vi "有效负载布放与回收.vi"() -> ()   [LabVIEW 2018]
uses:
  D:/Labview2018/examples/Instrument IO/Serial/support/Serial - Settings.ctl
  <vilib>/Instr/_visa.llb/VISA Configure Serial Port (Instr).vi
  <vilib>/Utility/inputDevices.llb/closeJoystick.vi
panel:
  in  "选项卡控件 8":T1(tab)
  out "潜航器模式":i32
  out "潜航器速度":i32
  out "悬停":bool
  out "定深":bool
  out "定向":bool
  in  "VISA资源名称":refnum<visa-resource-name>="COM1"
  in  "串口设置":T2={"波特率"=9600, "数据位"=8, "校验"=enum."None", "停止位"=10, "流控制"=0} {"流控制" items=["无"=0, "XON/XOFF"=1, "RTS/CTS"=2, "DTR/DSR"=4]; "停止位" items=["1.0"=10, "1.5"=15, "2.0"=20]; "数据位" min=5 max=8 step=1; "波特率" items=["75"=75, "110"=110, "134"=134, "150"=150, "300"=300, "600"=600, "1200"=1200, "1800"=1800, "2400"=2400, "4800"=4800, "7200"=7200, "9600"=9600, "14400"=14400, "19200"=19200, "28800"=28800, "38400"=38400, "56000"=56000, "57600"=57600, "115200"=115200, "128000"=128000, "230400"=230400]}
  out "指示灯":cluster{bool, bool, bool}
  out "位置信息":cluster{dbl, dbl}
  out "Polar Plot":picture caption="极坐标图"
  out "显示界面":T3
  out "桅杆升到位":bool
  out "桅杆降到位":bool
  out "挡板缸":bool
  out "俯仰缸":bool
  out "升降桅杆缸":bool
  out "仰到位":bool
  out "俯到位":bool
  out "挡板张开到位":bool
  out "挡板合拢到位":bool
  in  "停止":bool
  out "俯仰位移传感器":i64 caption="Output Value"
  out "挡板推进传感器":i64 caption="Output Value"
  out "升降桅杆位移传感器":i64 caption="Output Value"
  out "系统通讯故障":bool
  out "系统通讯正常":bool
  in  "照明灯":bool
  in  "停止 2":bool
  in  "抱紧 2":bool
  in  "打开 2":bool
  out "推进模块故障":bool caption="地位正常运行"
  out "推进模块正常":bool
  out "推进模块故障信息":string
  out "电机运行状态":bool
  out "未到位":bool
  out "缩回到位":bool
  out "推进到位":bool
  out "Output Value 18":dbl caption="Output Value" format="%.2f"
  out "Output Value 17":dbl caption="Output Value" format="%.2f"
  out "Output Value 16":dbl caption="Output Value" format="%.2f"
  out "Output Value 15":dbl caption="Output Value" format="%.2f"
  out "Output Value 14":dbl caption="Output Value" format="%.2f"
  out "Output Value 13":dbl caption="Output Value" format="%.2f"
  out "Output Value 12":dbl caption="Output Value" format="%.2f"
  out "Output Value 11":dbl caption="Output Value" format="%.2f"
  out "Output Value 10":dbl caption="Output Value" format="%.2f"
  out "Output Value 9":dbl caption="Output Value" format="%.2f"
  out "Output Value 8":dbl caption="Output Value" format="%.2f"
  out "Output Value 7":dbl caption="Output Value" format="%.2f"
  out "Output Value 6":dbl caption="Output Value" format="%.2f"
  out "Output Value 5":dbl caption="Output Value" format="%.2f"
  out "Output Value 4":dbl caption="Output Value" format="%.2f"
  out "Output Value 3":dbl caption="Output Value" format="%.2f"
  out "Output Value 2":dbl caption="Output Value" format="%.2f"
  out "Output Value":dbl format="%.2f"
  in  "Application filename":string="canceshi1"
  in  "IP Port":string="22222"
  in  "IP Address":string="192.168.0.10"
  out "旋转":dbl caption="Output Value" format="%.2f"
  out "升降":dbl caption="Output Value" format="%.2f"
  out "抱爪1":dbl caption="Output Value" format="%.2f"
  out "伺服阀":dbl caption="Output Value" format="%.2f"
  in  "停止":bool
  in  "抱紧":bool
  in  "打开":bool
  out "电机2运行状态":bool
  out "抱爪2未到位":bool
  out "抱爪2抱紧到位":bool
  out "抱爪2打开到位":bool
  out "电机1运行状态":bool
  out "抱爪1未到位":bool
  out "抱爪1抱紧到位":bool
  out "抱爪1打开到位":bool
  out "电机2或驱动器2故障":bool
  out "电机2或驱动器2正常":bool
  out "电机1或驱动器1故障":bool
  out "电机1或驱动器1正常":bool
  out "回转故障信息":string
  in  "停止 3":bool
  in  "原始位":bool
  in  "工作位":bool
  out "到达工作位":bool
  out "电机运行状态":bool
  out "未到位":bool
  out "到达原始位":bool
  out "回转模块故障":bool caption="地位正常运行"
  out "回转模块正常":bool
  # "单位/mm"
  # "单位/mm"
  # "单位/mm"
  # "推进控制模块"
  # "捕获臂控制模块"
  # "回转控制模块"
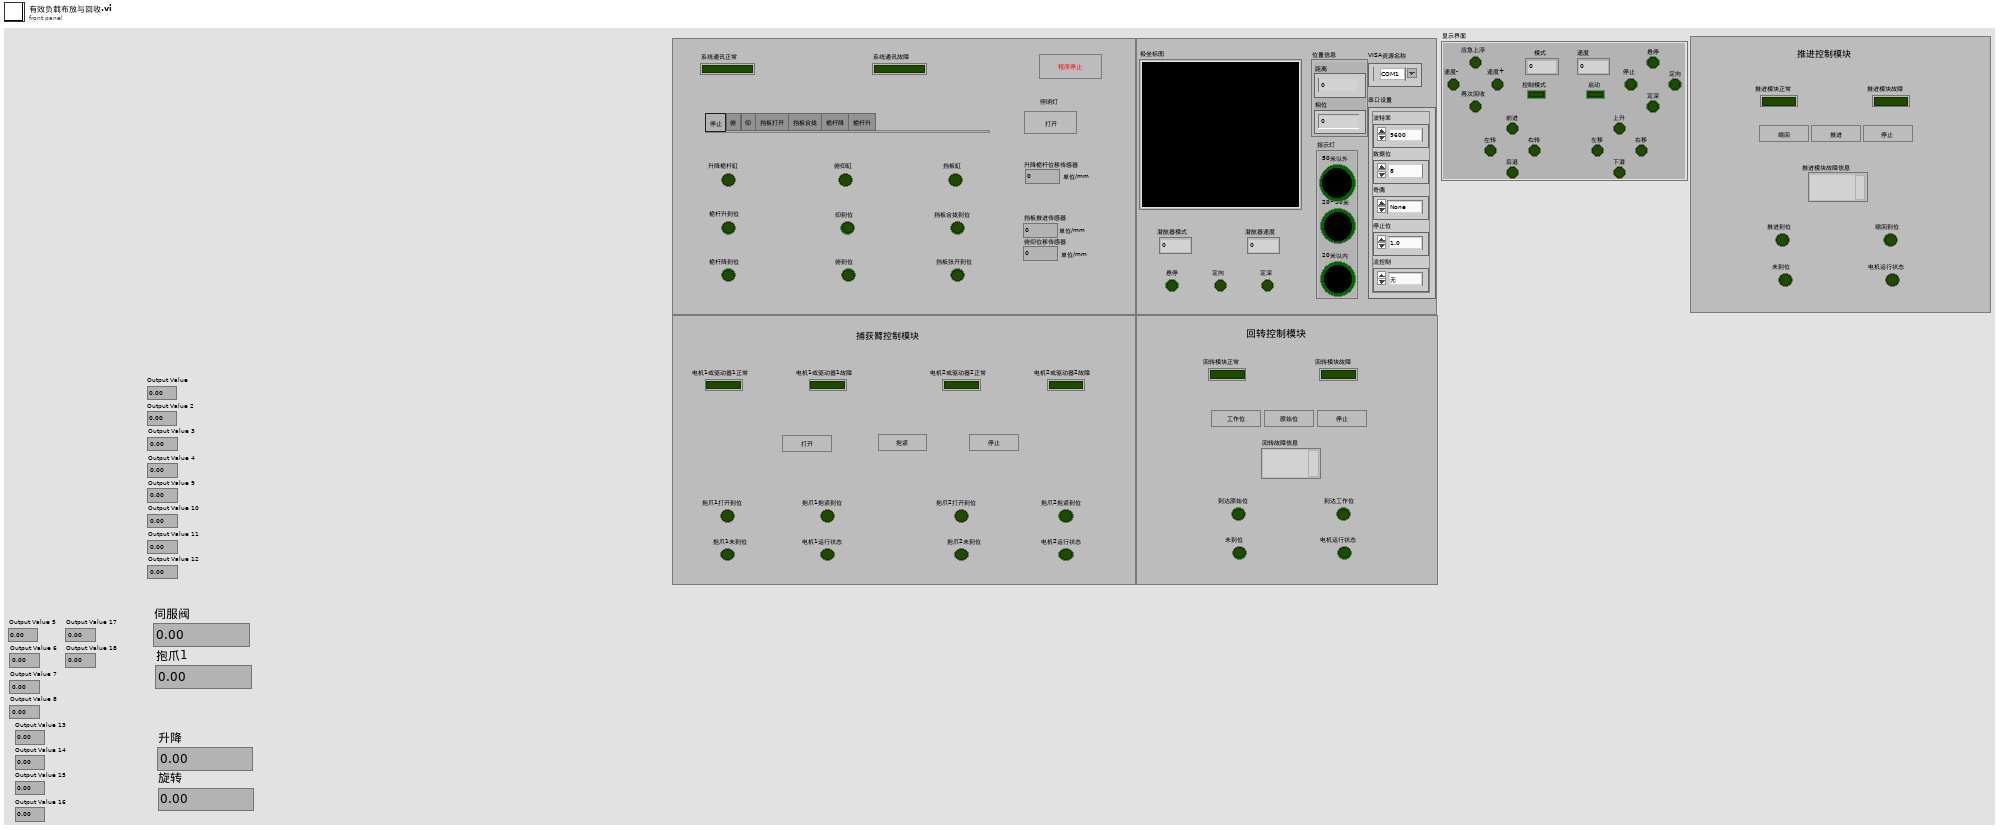
[diagram p1: front panel]
types:
  T1 = enum32{"停止", "俯", "仰", "挡板打开", "挡板合拢", "桅杆降", "桅杆升"}
  T2 = typedef "Serial - Settings.ctl" = cluster{"波特率":u32, "数据位":u16, "校验":enum16{"None", "Odd", "Even", "Mark", "Space"}, "停止位":u16, "流控制":u16}
  T3 = cluster{"右转":bool, "左转":bool, "后退":bool, "前进":bool, "右移":bool, "左移":bool, "下潜":bool, "上升":bool, "定深":bool, "定向":bool, "停止":bool, "悬停":bool, "控制模式":bool, "启动":bool, "应急上浮":bool, "再次回收":bool, "速度+":bool, "速度-":bool, "模式":i32, "速度":i32}
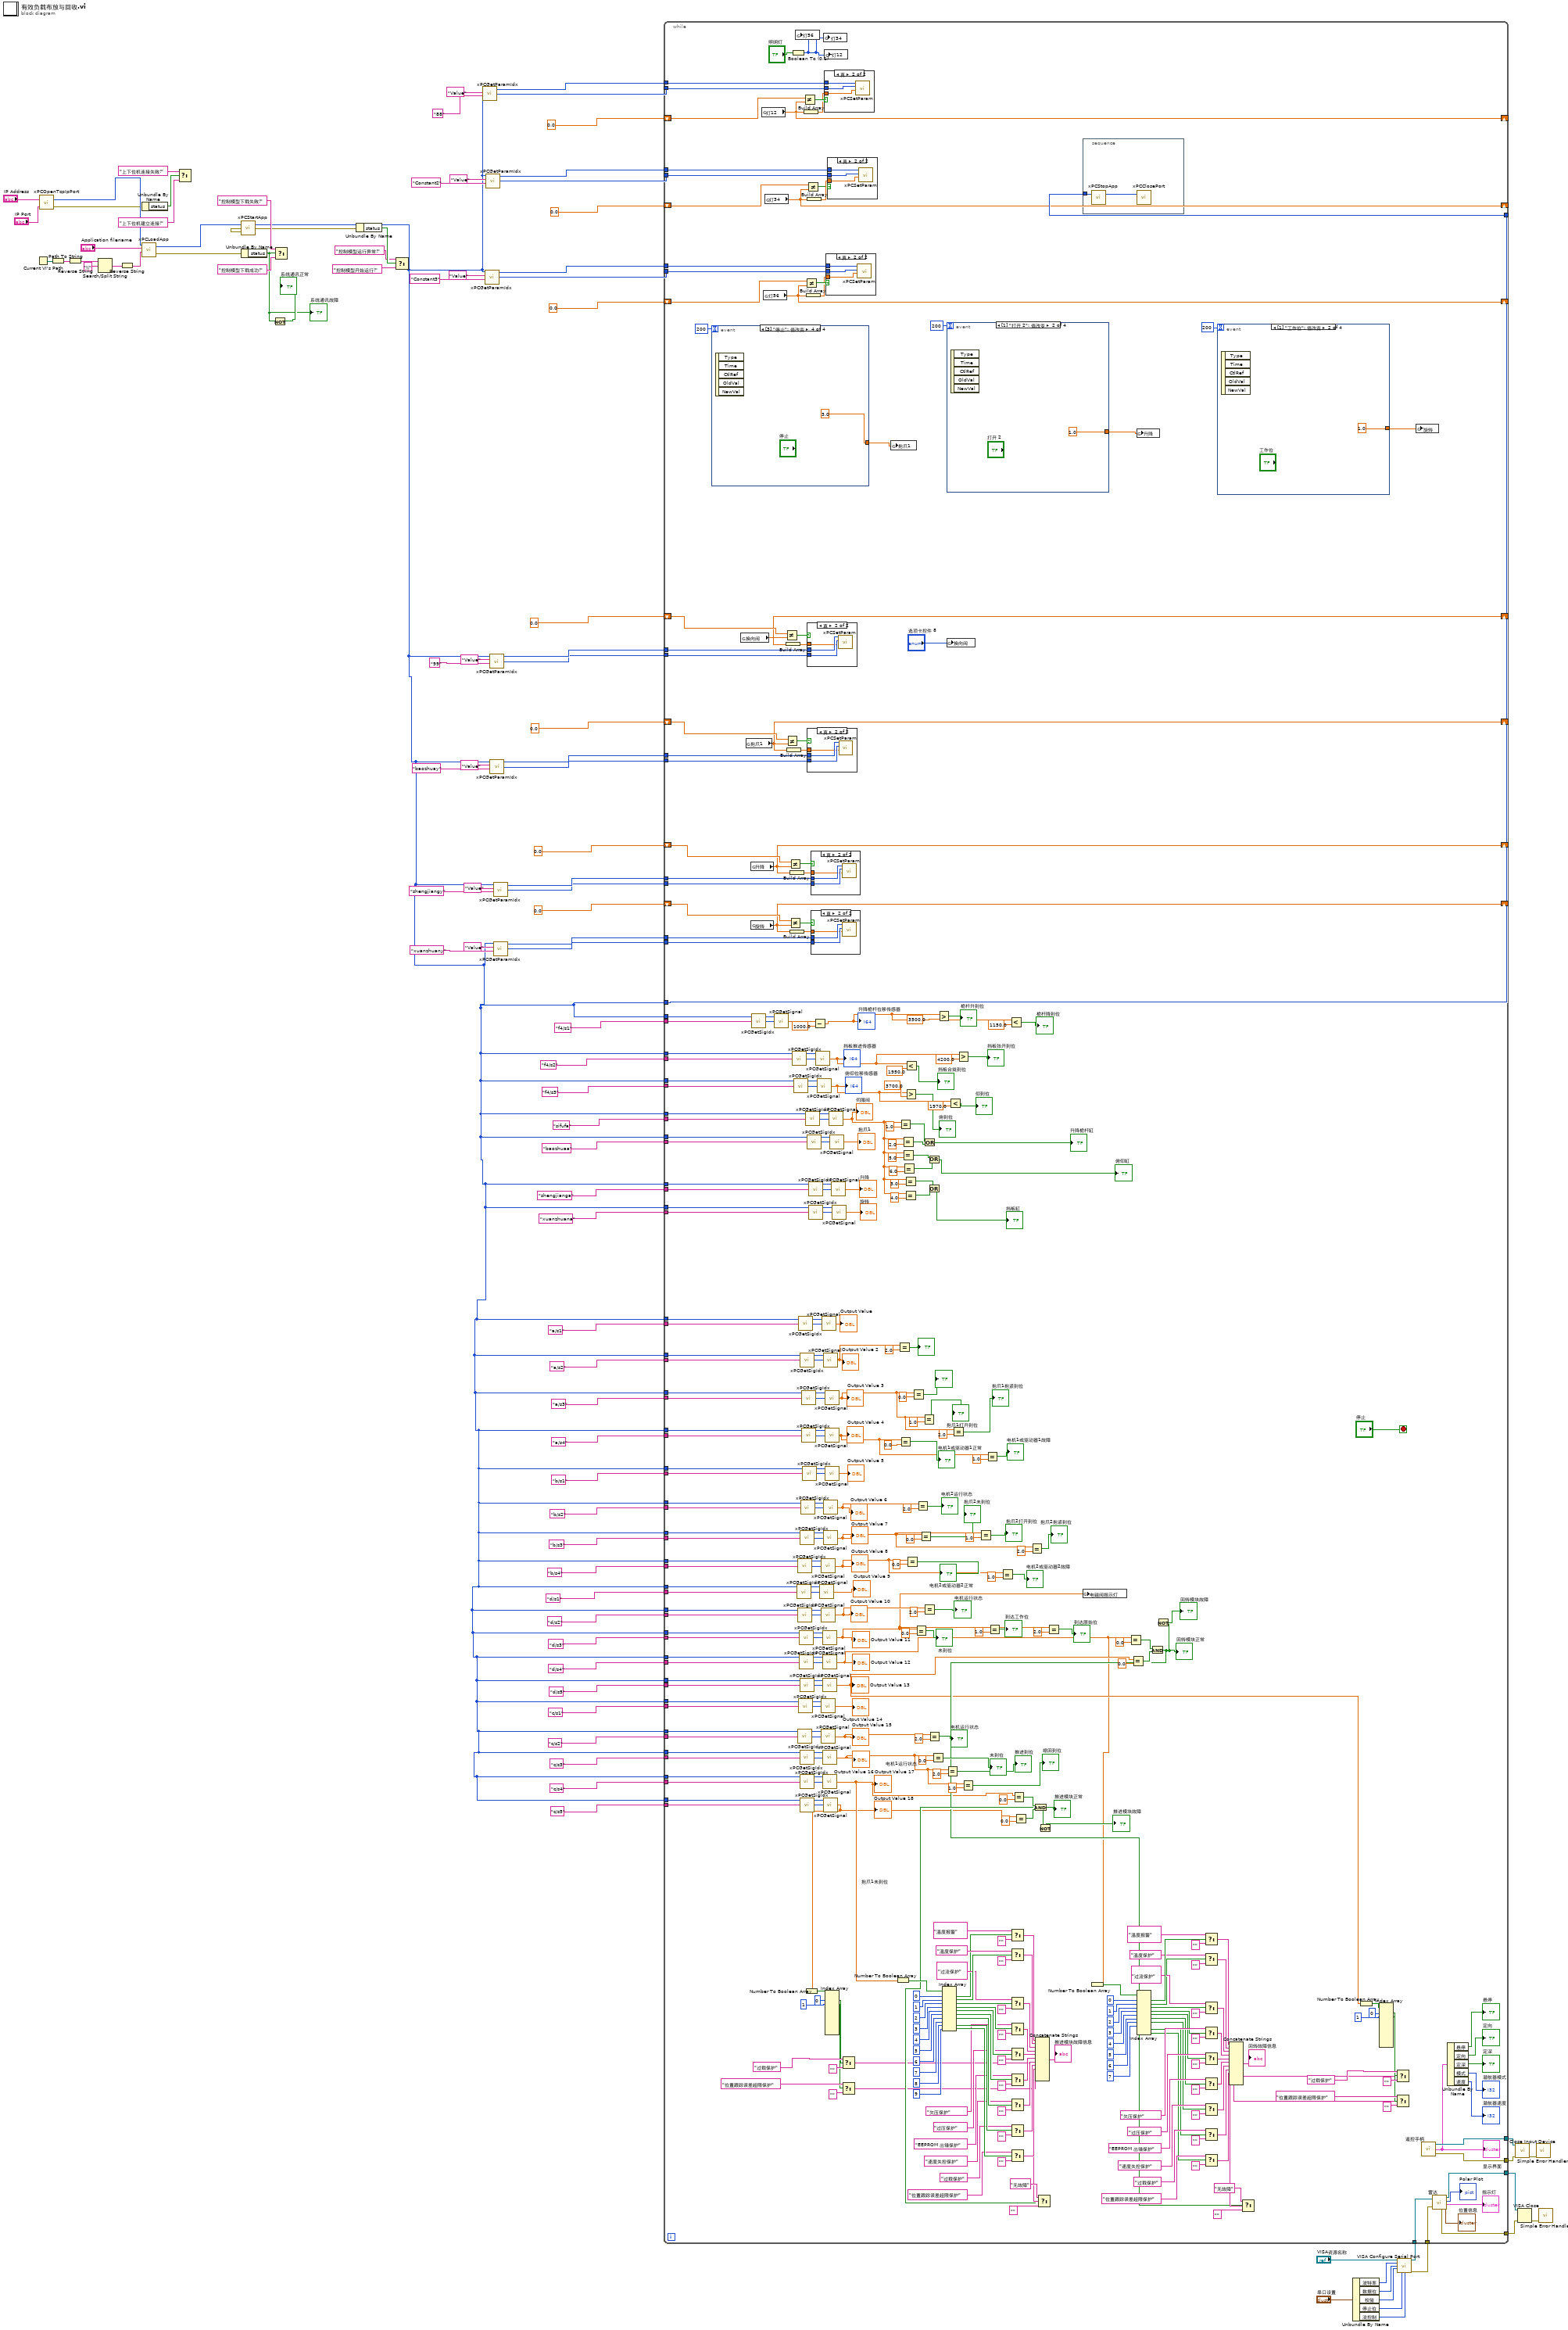
[diagram p0: block diagram]
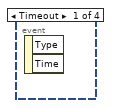
[diagram p2: hidden frame]
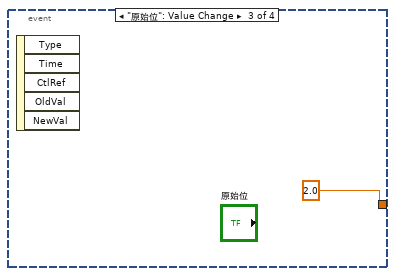
[diagram p3: hidden frame]
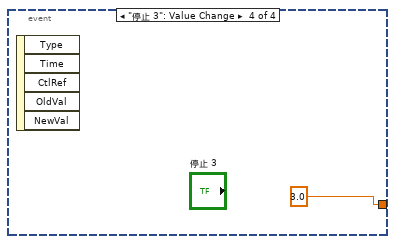
[diagram p4: hidden frame]
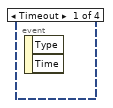
[diagram p5: hidden frame]
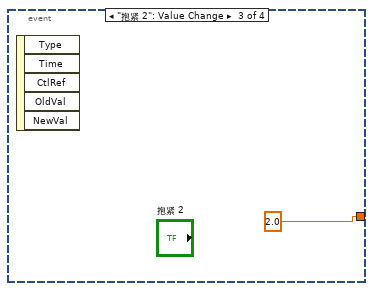
[diagram p6: hidden frame]
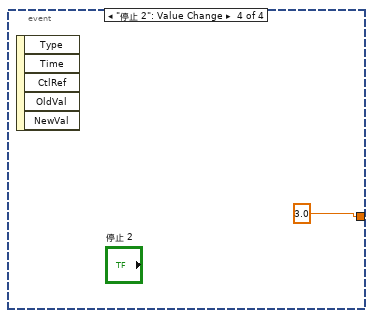
[diagram p7: hidden frame]
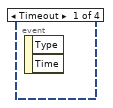
[diagram p8: hidden frame]
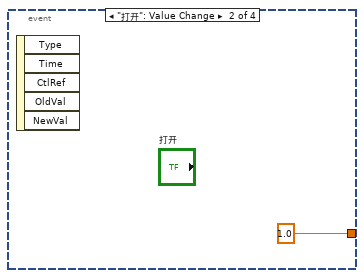
[diagram p9: hidden frame]
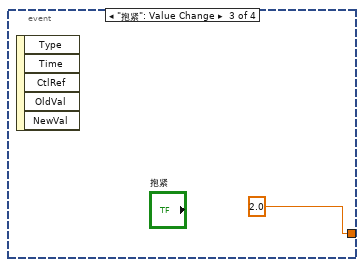
[diagram p10: hidden frame]
diagram:
  n1 = Current VI's Path() -> (path=w95:path)
  n2 = call "xPCOpenTcpIpPort.vi"("port"="IP Port", "address"="IP Address") -> ("error out"=w85:errorcluster, "Port"=w86:i32)
  n3 = Path To String(path=w95) -> (string=w97:string)
  n4 = Reverse String(1:w97) -> (0:w99:string)
  n5 = Search/Split String(string=w99, search string/char (-)="\\" ("search char (-)")) -> (match + rest of string=w98:string)  [unwired: 1 in, 2 out]
  n6 = Reverse String(1:w98) -> (0:w100:string)
  n7 = Unbundle By Name(w85) -> ("status"=w92:bool)
  n8 = call "xPCLoadApp.vi"("pathstr"=w100, "filename"="Application filename", "port"=w86) -> ("error out"=w87:errorcluster, "port copy"=w94:i32)  [unwired: 1 in]
  n9 = Select(t="上下位机连接失败!" ("message"), s=w92, f="上下位机建立连接!" ("message")) -> ()  [unwired: 1 out]
  n10 = call "xPCStartApp.vi"("port"=w94) -> ("error out"=w79:errorcluster, "port copy"=w16:i32)  [unwired: 1 in]
  n11 = Unbundle By Name(w87) -> ("status"=w52:bool)
  "系统通讯故障" <- w52
  n12 = Not(x=w52) -> (.not. x?=→"系统通讯正常":bool)
  n13 = Select(t="控制模型下载失败!" ("message"), s=w52, f="控制模型下载成功!" ("message")) -> ()  [unwired: 1 out]
  n14 = Unbundle By Name(w79) -> ("status"=w81:bool)
  n15 = Select(t="控制模型运行异常!" ("message"), s=w81, f="控制模型开始运行!" ("message")) -> ()  [unwired: 1 out]
  n16 = call "xPCGetParamIdx.vi"("blockpath"="88" ("pathstr"), "parametername"="Value" ("filename"), "port"=w16) -> ("identifier"=w72:i32, "port copy"=w73:i32)  [unwired: 1 in, 1 out]
  n17 = call "xPCGetParamIdx.vi"("blockpath"="Constant3" ("pathstr"), "parametername"="Value" ("filename"), "port"=w16) -> ("identifier"=w61:i32, "port copy"=w62:i32)  [unwired: 1 in, 1 out]
  n18 = call "xPCGetParamIdx.vi"("blockpath"="Constant2" ("pathstr"), "parametername"="Value" ("filename"), "port"=w16) -> ("identifier"=w66:i32, "port copy"=w65:i32)  [unwired: 1 in, 1 out]
  n19 = call "xPCGetParamIdx.vi"("blockpath"="99" ("pathstr"), "parametername"="Value" ("filename"), "port"=w16) -> ("identifier"=w58:i32, "port copy"=w76:i32)  [unwired: 1 in, 1 out]
  n20 = call "xPCGetParamIdx.vi"("blockpath"="baozhuay" ("pathstr"), "parametername"="Value" ("filename"), "port"=w16) -> ("identifier"=w31:i32, "port copy"=w29:i32)  [unwired: 1 in, 1 out]
  n21 = call "xPCGetParamIdx.vi"("blockpath"="shengjiangy" ("pathstr"), "parametername"="Value" ("filename"), "port"=w16) -> ("identifier"=w22:i32, "port copy"=w24:i32)  [unwired: 1 in, 1 out]
  n22 = call "xPCGetParamIdx.vi"("blockpath"="xuanzhuany" ("pathstr"), "parametername"="Value" ("filename"), "port"=w16) -> ("identifier"=w21:i32, "port copy"=w19:i32)  [unwired: 1 in, 1 out]
  n23 = Unbundle By Name("串口设置") -> ("波特率"=w7:u32, "数据位"=w8:u16, "校验"=w9:enum16{"None", "Odd", "Even", "Mark", "Space"}, "停止位"=w10:u16, "流控制"=w5:u16)
  n24 = call-poly "VISA Configure Serial Port"("VISA resource name"="VISA资源名称", "baud rate (9600)"=w7, "data bits (8)"=w8, "parity (0:none)"=w9, "stop bits (10: 1 bit)"=w10, "flow control (0:none)"=w5) -> ("VISA resource name out"=w4:refnum<visa-resource-name>, "error out"=w3:errorcluster)  [unwired: 4 in, 4 out]
  n25 = while {
    tunnel: w16 -> [w497]
    tunnel: [w497] -> w93
    shift-right: [w491] -> _
    shift-left: 0.0 -> [w494]
    tunnel: w58 -> [w493]
    tunnel: w76 -> [w492]
    shift-right: [w490] -> _
    shift-left: 0.0 -> [w489]
    tunnel: w72 -> [w486]
    tunnel: w73 -> [w485]
    tunnel: w16 -> [w483]
    tunnel: "f4/s1" ("pathstr") -> [w481]
    shift-right: [w474] -> _
    shift-left: 0.0 -> [w475]
    tunnel: w66 -> [w478]
    tunnel: w65 -> [w479]
    shift-right: [w473] -> _
    shift-left: 0.0 -> [w472]
    tunnel: w61 -> [w469]
    tunnel: w62 -> [w468]
    tunnel: w16 -> [w464]
    tunnel: "sifufa" ("pathstr") -> [w466]
    tunnel: w16 -> [w463]
    tunnel: "baozhuaa" ("pathstr") -> [w460]
    tunnel: w16 -> [w458]
    tunnel: "shengjianga" ("pathstr") -> [w455]
    tunnel: w16 -> [w449]
    tunnel: "xuanzhuana" ("pathstr") -> [w452]
    tunnel: w16 -> [w424]
    tunnel: "a/s1" ("pathstr") -> [w422]
    tunnel: w16 -> [w425]
    tunnel: "a/s2" ("pathstr") -> [w427]
    tunnel: w16 -> [w432]
    tunnel: "a/s3" ("pathstr") -> [w430]
    tunnel: w16 -> [w433]
    tunnel: "a/s4" ("pathstr") -> [w435]
    tunnel: w16 -> [w440]
    tunnel: "b/s1" ("pathstr") -> [w438]
    tunnel: w16 -> [w441]
    tunnel: "b/s2" ("pathstr") -> [w443]
    tunnel: w16 -> [w448]
    tunnel: "b/s3" ("pathstr") -> [w446]
    tunnel: w16 -> [w420]
    tunnel: "b/s4" ("pathstr") -> [w418]
    tunnel: w16 -> [w413]
    tunnel: "d/s1" ("pathstr") -> [w415]
    tunnel: w16 -> [w412]
    tunnel: "d/s2" ("pathstr") -> [w410]
    tunnel: w16 -> [w405]
    tunnel: "d/s3" ("pathstr") -> [w407]
    tunnel: w16 -> [w404]
    tunnel: "d/s4" ("pathstr") -> [w402]
    tunnel: w16 -> [w397]
    tunnel: "d/s5" ("pathstr") -> [w399]
    tunnel: w16 -> [w396]
    tunnel: "c/s1" ("pathstr") -> [w394]
    tunnel: w16 -> [w389]
    tunnel: "c/s2" ("pathstr") -> [w391]
    tunnel: w16 -> [w380]
    tunnel: "c/s3" ("pathstr") -> [w378]
    tunnel: w16 -> [w381]
    tunnel: "c/s4" ("pathstr") -> [w383]
    tunnel: w16 -> [w388]
    tunnel: "c/s5" ("pathstr") -> [w386]
    tunnel: w16 -> [w220]
    tunnel: "f4/s2" ("pathstr") -> [w222]
    tunnel: w16 -> [w219]
    tunnel: "f4/s3" ("pathstr") -> [w217]
    shift-right: [w161] -> _
    shift-left: 0.0 -> [w174]
    tunnel: w31 -> [w175]
    tunnel: w29 -> [w176]
    shift-right: [w160] -> _
    shift-left: 0.0 -> [w169]
    tunnel: w22 -> [w168]
    tunnel: w24 -> [w167]
    shift-right: [w159] -> _
    shift-left: 0.0 -> [w164]
    tunnel: w21 -> [w165]
    tunnel: w19 -> [w166]
    tunnel: [w117] -> w14
    tunnel: [w116] -> w13
    tunnel: w4 -> [w112]
    tunnel: w3 -> [w111]
    tunnel: [w110] -> w2
    tunnel: [w109] -> w1
    stop <- "停止" stop-if-true
    n26 = event shown="[3] \"停止\": 值改变" {
      selector: _ -> [_ _ _ _]
      dyn-events: _ -> [_ _ _ _]
      timeout: 200 -> [_ _ _ _]
      tunnel: [_ 1.0 ("抱爪1") 2.0 ("抱爪1") 3.0 ("抱爪1")] -> w157
      event Timeout {
        n27 = event-data() -> ()  [unwired: 1 in, 2 out]
      }
      event "打开": Value Change {
        n28 = event-data() -> ()  [unwired: 1 in, 5 out]
      }
      event "抱紧": Value Change {
        n29 = event-data() -> ()  [unwired: 1 in, 5 out]
      }
      event "停止": Value Change {
        n30 = event-data() -> ()  [unwired: 1 in, 5 out]
      }
    }
    n31 = global read "全局 1.vi" "换向阀"() -> (w491:dbl)
    n32 = global read "全局 1.vi" "抱爪1"() -> (w161:dbl)
    n33 = global read "全局 1.vi" "升降"() -> (w160:dbl)
    n34 = global read "全局 1.vi" "旋转"() -> (w159:dbl)
    n35 = call "xPCGetSigIdx.vi"("blockpath"=w481, "port"=w483) -> ("identifier"=w480:i32, "port copy"=w482:i32)  [unwired: 1 in, 1 out]
    n36 = global read "全局 1.vi" "灯12"() -> (w490:dbl)
    n37 = global read "全局 1.vi" "灯56"() -> (w473:dbl)
    n38 = global read "全局 1.vi" "灯34"() -> (w474:dbl)
    n39 = call "xPCGetSignal.vi"("signal"=w480, "port"=w482) -> ("Output Value"=w120:dbl)  [unwired: 1 in, 2 out]
    n40 = Not Equal?(x=w494, y=w491) -> (x != y?=w495:bool)
    n41 = Not Equal?(x=w174, y=w161) -> (x != y?=w173:bool)
    n42 = Build Array(w491) -> (w496:dbl[])
    n43 = Build Array(w161) -> (w172:dbl[])
    n44 = Not Equal?(x=w169, y=w160) -> (x != y?=w170:bool)
    n45 = Not Equal?(x=w164, y=w159) -> (x != y?=w163:bool)
    n46 = Build Array(w160) -> (w171:dbl[])
    n47 = Build Array(w159) -> (w162:dbl[])
    n48 = Boolean To (0,1)(Boolean="照明灯") -> (0, 1=w121:i16)
    n49 = call "xPCGetSigIdx.vi"("blockpath"=w222, "port"=w220) -> ("identifier"=w223:i32, "port copy"=w221:i32)  [unwired: 1 in, 1 out]
    n50 = call "xPCGetSigIdx.vi"("blockpath"=w217, "port"=w219) -> ("identifier"=w216:i32, "port copy"=w218:i32)  [unwired: 1 in, 1 out]
    n51 = global write "全局 1.vi" "灯56"(w121) -> ()
    n52 = call "xPCGetSigIdx.vi"("blockpath"=w415, "port"=w413) -> ("identifier"=w416:i32, "port copy"=w414:i32)  [unwired: 1 in, 1 out]
    n53 = call "xPCGetSigIdx.vi"("blockpath"=w418, "port"=w420) -> ("identifier"=w417:i32, "port copy"=w419:i32)  [unwired: 1 in, 1 out]
    n54 = call "xPCGetSigIdx.vi"("blockpath"=w410, "port"=w412) -> ("identifier"=w409:i32, "port copy"=w411:i32)  [unwired: 1 in, 1 out]
    n55 = call "xPCGetSigIdx.vi"("blockpath"=w391, "port"=w389) -> ("identifier"=w392:i32, "port copy"=w390:i32)  [unwired: 1 in, 1 out]
    n56 = call "xPCGetSigIdx.vi"("blockpath"=w394, "port"=w396) -> ("identifier"=w393:i32, "port copy"=w395:i32)  [unwired: 1 in, 1 out]
    n57 = call "xPCGetSigIdx.vi"("blockpath"=w422, "port"=w424) -> ("identifier"=w421:i32, "port copy"=w423:i32)  [unwired: 1 in, 1 out]
    n58 = call "xPCGetSigIdx.vi"("blockpath"=w407, "port"=w405) -> ("identifier"=w408:i32, "port copy"=w406:i32)  [unwired: 1 in, 1 out]
    n59 = call "xPCGetSigIdx.vi"("blockpath"=w402, "port"=w404) -> ("identifier"=w401:i32, "port copy"=w403:i32)  [unwired: 1 in, 1 out]
    n60 = call "xPCGetSigIdx.vi"("blockpath"=w399, "port"=w397) -> ("identifier"=w400:i32, "port copy"=w398:i32)  [unwired: 1 in, 1 out]
    n61 = call "xPCGetSigIdx.vi"("blockpath"=w378, "port"=w380) -> ("identifier"=w377:i32, "port copy"=w379:i32)  [unwired: 1 in, 1 out]
    n62 = call "xPCGetSigIdx.vi"("blockpath"=w383, "port"=w381) -> ("identifier"=w384:i32, "port copy"=w382:i32)  [unwired: 1 in, 1 out]
    n63 = call "xPCGetSigIdx.vi"("blockpath"=w427, "port"=w425) -> ("identifier"=w428:i32, "port copy"=w426:i32)  [unwired: 1 in, 1 out]
    n64 = call "xPCGetSigIdx.vi"("blockpath"=w446, "port"=w448) -> ("identifier"=w445:i32, "port copy"=w447:i32)  [unwired: 1 in, 1 out]
    n65 = call "xPCGetSigIdx.vi"("blockpath"=w386, "port"=w388) -> ("identifier"=w385:i32, "port copy"=w387:i32)  [unwired: 1 in, 1 out]
    n66 = call "xPCGetSigIdx.vi"("blockpath"=w443, "port"=w441) -> ("identifier"=w444:i32, "port copy"=w442:i32)  [unwired: 1 in, 1 out]
    n67 = call "xPCGetSigIdx.vi"("blockpath"=w430, "port"=w432) -> ("identifier"=w429:i32, "port copy"=w431:i32)  [unwired: 1 in, 1 out]
    n68 = call "xPCGetSigIdx.vi"("blockpath"=w435, "port"=w433) -> ("identifier"=w436:i32, "port copy"=w434:i32)  [unwired: 1 in, 1 out]
    n69 = call "xPCGetSigIdx.vi"("blockpath"=w438, "port"=w440) -> ("identifier"=w437:i32, "port copy"=w439:i32)  [unwired: 1 in, 1 out]
    n70 = Not Equal?(x=w489, y=w490) -> (x != y?=w488:bool)
    n71 = Build Array(w490) -> (w487:dbl[])
    n72 = Not Equal?(x=w472, y=w473) -> (x != y?=w471:bool)
    n73 = call "xPCGetSigIdx.vi"("blockpath"=w466, "port"=w464) -> ("identifier"=w467:i32, "port copy"=w465:i32)  [unwired: 1 in, 1 out]
    n74 = Not Equal?(x=w475, y=w474) -> (x != y?=w476:bool)
    n75 = Build Array(w473) -> (w470:dbl[])
    n76 = case shown="真" w495 {
      tunnel: w492 -> [_ w527]
      tunnel: w493 -> [_ w526]
      tunnel: w496 -> [_ w525]
      frame False {
      }
      frame True {
        n77 = call "xPCSetParam.vi"("value"=w525, "index"=w526, "port"=w527) -> ()  [unwired: 1 in, 2 out]
      }
    }
    n78 = call "xPCGetSigIdx.vi"("blockpath"=w460, "port"=w463) -> ("identifier"=w459:i32, "port copy"=w462:i32)  [unwired: 1 in, 1 out]
    n79 = Build Array(w474) -> (w477:dbl[])
    n80 = case shown="真" w173 {
      tunnel: w176 -> [_ w515]
      tunnel: w175 -> [_ w514]
      tunnel: w172 -> [_ w513]
      frame False {
      }
      frame True {
        n81 = call "xPCSetParam.vi"("value"=w513, "index"=w514, "port"=w515) -> ()  [unwired: 1 in, 2 out]
      }
    }
    n82 = call "xPCGetSigIdx.vi"("blockpath"=w455, "port"=w458) -> ("identifier"=w454:i32, "port copy"=w457:i32)  [unwired: 1 in, 1 out]
    n83 = call "xPCGetSigIdx.vi"("blockpath"=w452, "port"=w449) -> ("identifier"=w453:i32, "port copy"=w450:i32)  [unwired: 1 in, 1 out]
    n84 = case shown="真" w170 {
      tunnel: w167 -> [_ w512]
      tunnel: w168 -> [_ w511]
      tunnel: w171 -> [_ w510]
      frame False {
      }
      frame True {
        n85 = call "xPCSetParam.vi"("value"=w510, "index"=w511, "port"=w512) -> ()  [unwired: 1 in, 2 out]
      }
    }
    n86 = case shown="真" w163 {
      tunnel: w166 -> [_ w509]
      tunnel: w165 -> [_ w508]
      tunnel: w162 -> [_ w507]
      frame False {
      }
      frame True {
        n87 = call "xPCSetParam.vi"("value"=w507, "index"=w508, "port"=w509) -> ()  [unwired: 1 in, 2 out]
      }
    }
    n88 = Subtract(x=w120, y=1000.0) -> (x-y=w118:dbl)
    "升降桅杆位移传感器" <- w118
    n89 = call "xPCGetSignal.vi"("signal"=w223, "port"=w221) -> ("Output Value"=w151:dbl)  [unwired: 1 in, 2 out]
    "挡板推进传感器" <- w151
    n90 = call "xPCGetSignal.vi"("signal"=w216, "port"=w218) -> ("Output Value"=w145:dbl)  [unwired: 1 in, 2 out]
    "俯仰位移传感器" <- w145
    n91 = call "xPCGetSignal.vi"("signal"=w416, "port"=w414) -> ("Output Value"=→"Output Value 9":dbl)  [unwired: 1 in, 2 out]
    n92 = call "xPCGetSignal.vi"("signal"=w417, "port"=w419) -> ("Output Value"=w344:dbl)  [unwired: 1 in, 2 out]
    "Output Value 8" <- w344
    n93 = call "xPCGetSignal.vi"("signal"=w409, "port"=w411) -> ("Output Value"=w341:dbl)  [unwired: 1 in, 2 out]
    "Output Value 10" <- w341
    n94 = call "xPCGetSignal.vi"("signal"=w392, "port"=w390) -> ("Output Value"=w331:dbl)  [unwired: 1 in, 2 out]
    "Output Value 15" <- w331
    n95 = call "xPCGetSignal.vi"("signal"=w393, "port"=w395) -> ("Output Value"=→"Output Value 14":dbl)  [unwired: 1 in, 2 out]
    n96 = call "xPCGetSignal.vi"("signal"=w421, "port"=w423) -> ("Output Value"=→"Output Value":dbl)  [unwired: 1 in, 2 out]
    n97 = call "xPCGetSignal.vi"("signal"=w408, "port"=w406) -> ("Output Value"=w125:dbl)  [unwired: 1 in, 2 out]
    "Output Value 11" <- w125
    n98 = call "xPCGetSignal.vi"("signal"=w401, "port"=w403) -> ("Output Value"=w177:dbl)  [unwired: 1 in, 2 out]
    "Output Value 12" <- w177
    n99 = call "xPCGetSignal.vi"("signal"=w400, "port"=w398) -> ("Output Value"=w182:dbl)  [unwired: 1 in, 2 out]
    "Output Value 13" <- w182
    n100 = call "xPCGetSignal.vi"("signal"=w377, "port"=w379) -> ("Output Value"=w324:dbl)  [unwired: 1 in, 2 out]
    "Output Value 16" <- w324
    n101 = call "xPCGetSignal.vi"("signal"=w384, "port"=w382) -> ("Output Value"=w195:dbl)  [unwired: 1 in, 2 out]
    "Output Value 17" <- w195
    n102 = global write "全局 1.vi" "灯34"(w121) -> ()
    n103 = call "xPCGetSignal.vi"("signal"=w428, "port"=w426) -> ("Output Value"=w371:dbl)  [unwired: 1 in, 2 out]
    "Output Value 2" <- w371
    n104 = call "xPCGetSignal.vi"("signal"=w445, "port"=w447) -> ("Output Value"=w346:dbl)  [unwired: 1 in, 2 out]
    "Output Value 7" <- w346
    n105 = call "xPCGetSignal.vi"("signal"=w385, "port"=w387) -> ("Output Value"=w194:dbl)  [unwired: 1 in, 2 out]
    "Output Value 18" <- w194
    n106 = Number To Boolean Array(number=w194) -> (Boolean array=w196:bool[])
    n107 = call "xPCGetSignal.vi"("signal"=w444, "port"=w442) -> ("Output Value"=w353:dbl)  [unwired: 1 in, 2 out]
    "Output Value 6" <- w353
    n108 = global write "全局 1.vi" "灯12"(w121) -> ()
    n109 = case shown="真" w488 {
      tunnel: w487 -> [_ w524]
      tunnel: w486 -> [_ w523]
      tunnel: w485 -> [_ w522]
      frame False {
      }
      frame True {
        n110 = call "xPCSetParam.vi"("value"=w524, "index"=w523, "port"=w522) -> ()  [unwired: 1 in, 2 out]
      }
    }
    n111 = call "xPCGetSignal.vi"("signal"=w429, "port"=w431) -> ("Output Value"=w365:dbl)  [unwired: 1 in, 2 out]
    "Output Value 3" <- w365
    n112 = call "xPCGetSignal.vi"("signal"=w436, "port"=w434) -> ("Output Value"=w355:dbl)  [unwired: 1 in, 2 out]
    "Output Value 4" <- w355
    n113 = Index Array(array=w196, index #1=0 ("索引"), index #2=1 ("索引")) -> (element #1=w193:bool, element #2=w192:bool)  [unwired: 8 in, 8 out]
    n114 = call "xPCGetSignal.vi"("signal"=w437, "port"=w439) -> ("Output Value"=→"Output Value 5":dbl)  [unwired: 1 in, 2 out]
    n115 = case shown="真" w471 {
      tunnel: w470 -> [_ w518]
      tunnel: w469 -> [_ w517]
      tunnel: w468 -> [_ w516]
      frame False {
      }
      frame True {
        n116 = call "xPCSetParam.vi"("value"=w518, "index"=w517, "port"=w516) -> ()  [unwired: 1 in, 2 out]
      }
    }
    n117 = case shown="真" w476 {
      tunnel: w477 -> [_ w521]
      tunnel: w478 -> [_ w520]
      tunnel: w479 -> [_ w519]
      frame False {
      }
      frame True {
        n118 = call "xPCSetParam.vi"("value"=w521, "index"=w520, "port"=w519) -> ()  [unwired: 1 in, 2 out]
      }
    }
    n119 = call "xPCGetSignal.vi"("signal"=w467, "port"=w465) -> ("Output Value"=w136:dbl)  [unwired: 1 in, 2 out]
    "伺服阀" <- w136
    n120 = call "xPCGetSignal.vi"("signal"=w459, "port"=w462) -> ("Output Value"=→"抱爪1":dbl)  [unwired: 1 in, 2 out]
    n121 = call "xPCGetSignal.vi"("signal"=w454, "port"=w457) -> ("Output Value"=→"升降":dbl)  [unwired: 1 in, 2 out]
    n122 = call "xPCGetSignal.vi"("signal"=w453, "port"=w450) -> ("Output Value"=→"旋转":dbl)  [unwired: 1 in, 2 out]
    n123 = Select(t="过载保护" ("message"), s=w193, f="" ("message")) -> (s? t:f=w191:string)
    n124 = Select(t="位置跟踪误差超限保护" ("message"), s=w192, f="" ("message")) -> (s? t:f=w190:string)
    n125 = global write "全局 1.vi" "抱爪1"(w157) -> ()
    n126 = Number To Boolean Array(number=w195) -> (Boolean array=w281:bool[])
    n127 = Equal?(x=w371, y=2.0) -> (x = y?=→"电机1运行状态":bool)
    n128 = Equal?(x=w136, y=1.0) -> (x = y?=w135:bool)
    n129 = Equal?(x=w355, y=0.0) -> (x = y?=→"电机1或驱动器1正常":bool)
    n130 = Equal?(x=w136, y=2.0) -> (x = y?=w134:bool)
    n131 = Equal?(x=w136, y=5.0) -> (x = y?=w133:bool)
    n132 = Equal?(x=w136, y=6.0) -> (x = y?=w132:bool)
    n133 = Equal?(x=w136, y=3.0) -> (x = y?=w131:bool)
    n134 = Equal?(x=w136, y=4.0) -> (x = y?=w130:bool)
    n135 = Greater?(x=w145, y=3700.0) -> (0:→"俯到位":bool)
    n136 = Less?(x=w151, y=1950.0) -> (x < y?=→"挡板合拢到位":bool)
    n137 = Equal?(x=w344, y=0.0) -> (x = y?=→"电机2或驱动器2正常":bool)
    n138 = Equal?(x=w365, y=0.0) -> (x = y?=→"抱爪1未到位":bool)
    n139 = Equal?(x=w125, y=0.0) -> (x = y?=→"未到位":bool)
    n140 = Equal?(x=w353, y=2.0) -> (x = y?=→"电机2运行状态":bool)
    n141 = Equal?(x=w346, y=0.0) -> (x = y?=→"抱爪2未到位":bool)
    n142 = Equal?(x=w365, y=1.0) -> (x = y?=→"抱爪1打开到位":bool)
    n143 = Or(x=w135, y=w134) -> (x .or. y?=→"升降桅杆缸":bool)
    n144 = Equal?(x=w341, y=2.0) -> (x = y?=→"电机运行状态":bool)
    n145 = Or(x=w133, y=w132) -> (x .or. y?=→"俯仰缸":bool)
    n146 = Or(x=w131, y=w130) -> (x .or. y?=→"挡板缸":bool)
    n147 = Equal?(x=w331, y=2.0) -> (x = y?=→"电机运行状态":bool)
    n148 = Equal?(x=w324, y=0.0) -> (x = y?=→"未到位":bool)
    n149 = Greater?(x=w118, y=3500.0) -> (0:→"桅杆升到位":bool)
    n150 = Index Array(array=w281, index #1=0 ("索引"), index #2=1 ("索引"), index #3=2 ("索引"), index #4=3 ("索引"), index #5=4 ("索引"), index #6=5 ("索引"), index #7=6 ("索引"), index #8=7 ("索引"), index #9=8 ("索引"), index #10=9 ("索引")) -> (element #1=w283:bool, element #2=w306:bool, element #3=w289:bool, element #4=w292:bool, element #5=w294:bool, element #6=w302:bool, element #7=w313:bool, element #9=w314:bool, element #10=w315:bool)  [unwired: 1 out]
    n151 = Equal?(x=w324, y=2.0) -> (x = y?=→"推进到位":bool)
    n152 = global write "全局 1.vi" "换向阀"("选项卡控件 8") -> ()
    n153 = event shown="[1] \"打开 2\": 值改变" {
      selector: _ -> [_ _ _ _]
      dyn-events: _ -> [_ _ _ _]
      timeout: 200 -> [_ _ _ _]
      tunnel: [_ 1.0 ("抱爪1") 2.0 ("抱爪1") 3.0 ("抱爪1")] -> w156
      event Timeout {
        n154 = event-data() -> ()  [unwired: 1 in, 2 out]
      }
      event "打开 2": Value Change {
        n155 = event-data() -> ()  [unwired: 1 in, 5 out]
      }
      event "抱紧 2": Value Change {
        n156 = event-data() -> ()  [unwired: 1 in, 5 out]
      }
      event "停止 2": Value Change {
        n157 = event-data() -> ()  [unwired: 1 in, 5 out]
      }
    }
    n158 = Less?(x=w145, y=1970.0) -> (x < y?=→"仰到位":bool)
    n159 = Equal?(x=w365, y=2.0) -> (x = y?=→"抱爪1抱紧到位":bool)
    n160 = Greater?(x=w151, y=4200.0) -> (0:→"挡板张开到位":bool)
    n161 = Equal?(x=w324, y=1.0) -> (x = y?=→"缩回到位":bool)
    n162 = Equal?(x=w346, y=1.0) -> (x = y?=→"抱爪2打开到位":bool)
    n163 = Equal?(x=w355, y=1.0) -> (x = y?=→"电机1或驱动器1故障":bool)
    n164 = Equal?(x=w125, y=1.0) -> (x = y?=→"到达工作位":bool)
    n165 = Equal?(x=w344, y=1.0) -> (x = y?=→"电机2或驱动器2故障":bool)
    n166 = Less?(x=w118, y=1150.0) -> (x < y?=→"桅杆降到位":bool)
    n167 = Select(t="温度报警" ("message"), s=w283, f="" ("message")) -> (s? t:f=w295:string)
    n168 = Select(t="温度保护" ("message"), s=w306, f="" ("message")) -> (s? t:f=w296:string)
    n169 = Select(t="过流保护" ("message"), s=w289, f="" ("message")) -> (s? t:f=w297:string)
    n170 = Select(t="欠压保护" ("message"), s=w292, f="" ("message")) -> (s? t:f=w298:string)
    n171 = Select(t="过压保护" ("message"), s=w294, f="" ("message")) -> (s? t:f=w299:string)
    n172 = Select(t="EEPROM 出错保护" ("message"), s=w302, f="" ("message")) -> (s? t:f=w316:string)
    n173 = Select(t="速度失控保护" ("message"), s=w313, f="" ("message")) -> (s? t:f=w317:string)
    n174 = Select(t="过载保护" ("message"), s=w314, f="" ("message")) -> (s? t:f=w318:string)
    n175 = Select(t="位置跟踪误差超限保护" ("message"), s=w315, f="" ("message")) -> (s? t:f=w319:string)
    n176 = Equal?(x=w195, y=0.0) -> (x = y?=w212:bool)
    n177 = Equal?(x=w194, y=0.0) -> (x = y?=w211:bool)
    n178 = Equal?(x=w346, y=2.0) -> (x = y?=→"抱爪2抱紧到位":bool)
    n179 = And(x=w212, y=w211) -> (x .and. y?=w204:bool)
    "推进模块正常" <- w204
    n180 = Select(t="无故障" ("message"), s=w204, f="" ("message")) -> (s? t:f=w225:string)
    n181 = Concatenate Strings(w295, w296, w297, w298, w299, w316, w317, w318, w319, w225, w191, w190) -> (→"推进模块故障信息":string)
    n182 = Not(x=w204) -> (.not. x?=→"推进模块故障":bool)
    n183 = Equal?(x=w125, y=2.0) -> (x = y?=→"到达原始位":bool)
    n184 = global write "全局 1.vi" "电磁阀指示灯"(w125) -> ()
    n185 = Number To Boolean Array(number=w177) -> (Boolean array=w272:bool[])
    n186 = Equal?(x=w177, y=0.0) -> (x = y?=w208:bool)
    n187 = Equal?(x=w182, y=0.0) -> (x = y?=w209:bool)
    n188 = global write "全局 1.vi" "升降"(w156) -> ()
    n189 = Index Array(array=w272, index #1=0 ("索引"), index #2=1 ("索引"), index #3=2 ("索引"), index #4=3 ("索引"), index #5=4 ("索引"), index #6=5 ("索引"), index #7=6 ("索引"), index #8=7 ("索引")) -> (element #1=w270:bool, element #2=w247:bool, element #3=w264:bool, element #4=w261:bool, element #5=w259:bool, element #6=w251:bool, element #7=w242:bool, element #9=w241:bool, element #10=w240:bool)  [unwired: 2 in, 1 out]
    n190 = And(x=w208, y=w209) -> (x .and. y?=w203:bool)
    "回转模块正常" <- w203
    n191 = Not(x=w203) -> (.not. x?=→"回转模块故障":bool)
    n192 = Select(t="温度报警" ("message"), s=w270, f="" ("message")) -> (s? t:f=w258:string)
    n193 = Select(t="温度保护" ("message"), s=w247, f="" ("message")) -> (s? t:f=w257:string)
    n194 = Select(t="过流保护" ("message"), s=w264, f="" ("message")) -> (s? t:f=w256:string)
    n195 = Select(t="欠压保护" ("message"), s=w261, f="" ("message")) -> (s? t:f=w255:string)
    n196 = Select(t="过压保护" ("message"), s=w259, f="" ("message")) -> (s? t:f=w254:string)
    n197 = Select(t="EEPROM 出错保护" ("message"), s=w251, f="" ("message")) -> (s? t:f=w239:string)
    n198 = Select(t="速度失控保护" ("message"), s=w242, f="" ("message")) -> (s? t:f=w238:string)
    n199 = Select(t="过载保护" ("message"), s=w241, f="" ("message")) -> (s? t:f=w237:string)
    n200 = Select(t="位置跟踪误差超限保护" ("message"), s=w240, f="" ("message")) -> (s? t:f=w236:string)
    n201 = event shown="[1] \"工作位\": 值改变" {
      selector: _ -> [_ _ _ _]
      dyn-events: _ -> [_ _ _ _]
      timeout: 200 -> [_ _ _ _]
      tunnel: [_ 1.0 ("抱爪1") 2.0 ("抱爪1") 3.0 ("抱爪1")] -> w155
      event Timeout {
        n202 = event-data() -> ()  [unwired: 1 in, 2 out]
      }
      event "工作位": Value Change {
        n203 = event-data() -> ()  [unwired: 1 in, 5 out]
      }
      event "原始位": Value Change {
        n204 = event-data() -> ()  [unwired: 1 in, 5 out]
      }
      event "停止 3": Value Change {
        n205 = event-data() -> ()  [unwired: 1 in, 5 out]
      }
    }
    n206 = Select(t="无故障" ("message"), s=w203, f="" ("message")) -> (s? t:f=w224:string)
    n207 = Number To Boolean Array(number=w182) -> (Boolean array=w183:bool[])
    n208 = Index Array(array=w183, index #1=0 ("索引"), index #2=1 ("索引")) -> (element #1=w181:bool, element #2=w180:bool)  [unwired: 8 in, 8 out]
    n209 = Select(t="过载保护" ("message"), s=w181, f="" ("message")) -> (s? t:f=w179:string)
    n210 = Select(t="位置跟踪误差超限保护" ("message"), s=w180, f="" ("message")) -> (s? t:f=w178:string)
    n211 = Concatenate Strings(w258, w257, w256, w255, w254, w239, w238, w237, w236, w224, w179, w178) -> (→"回转故障信息":string)
    n212 = global write "全局 1.vi" "旋转"(w155) -> ()
    n213 = call "遥控手柄.vi"() -> ("error out"=w116:errorcluster, "显示界面"=w107:T3, "device ID"=w117:refnum<k1>)
    "显示界面" <- w107
    n214 = call "雷达.vi"("错误输入（无错误）"=w111, "VISA资源名称"=w112) -> ("位置信息"=→"位置信息":cluster{dbl, dbl}, "指示灯"=→"指示灯":cluster{bool, bool, bool}, "Polar Plot"=→"Polar Plot":picture, "VISA资源名称输出"=w110:refnum<visa-resource-name>, "错误输出"=w109:errorcluster)
    n215 = Unbundle By Name(w107) -> ("悬停"=→"悬停":bool, "定向"=→"定向":bool, "定深"=→"定深":bool, "模式"=→"潜航器模式":i32, "速度"=→"潜航器速度":i32)
  }
  n216 = stacked-sequence {
    tunnel: w93 -> [w528]
    frame #0 {
      n217 = call "xPCStopApp.vi"("port"=w528) -> ("port copy"=w529:i32)  [unwired: 1 in, 1 out]
      n218 = call "xPCClosePort.vi"("port"=w529) -> ()  [unwired: 1 in, 2 out]
    }
  }
  n219 = call-poly <vilib>:"Close Input Device.vi"("error in (no error)"=w13, "device ID"=w14) -> ("error out"=w15:errorcluster)  [unwired: 8 in]
  n220 = VISA Close(VISA resource name=w2, error in (no error)=w1) -> (error out=w12:errorcluster)
  n221 = call <vilib>:"Simple Error Handler.vi"("error in (no error)"=w15) -> ()  [unwired: 4 in, 5 out]
  n222 = call <vilib>:"Simple Error Handler.vi"("error in (no error)"=w12) -> ()  [unwired: 1 in, 8 out]
